vi "DMM Configuration - Update DMM Controls Items.vi"(6 "Measurement In":T2 caption="Function", 7 "Resolution in Digits Saved Value":dbl, 8 "error in (no error)":errorcluster, 11 "Measurement Controls Refs":T1) -> (0 "error out":errorcluster, 1 "Resolution in Digits Array Out":dbl[](array[numeric]), 2 "Resolution in Digits Index":i32)   [LabVIEW 2016, in "DMM-SWITCH-ScanList System Explorer.lvlib"]
doc: "Measurements, Range and Resolution in Digits original type definitions from the DMM driver were very old controls. In order to use System Controls to match our Custom Device guidelines this VI was necessary to populate the new System Controls with the data from the original Type Definitions."
uses:
  DMM-SWITCH-ScanList System Explorer.lvlib
  <instrlib>/niDMM/nidmm.llb/niDMM Resolution in Digits.ctl
  <instrlib>/niDMM/nidmm.llb/niDMM Function.ctl
panel:
  in  "Measurement Type Def":T2 caption="Function"
  in  "Resolution in Digits Type Def":T3=6.5 caption="Resolution In Digits Type Def" items=["3 1/2"=3.5, "4 1/2"=4.5, "5 1/2"=5.5, "6 1/2"=6.5, "7 1/2"=7.5]
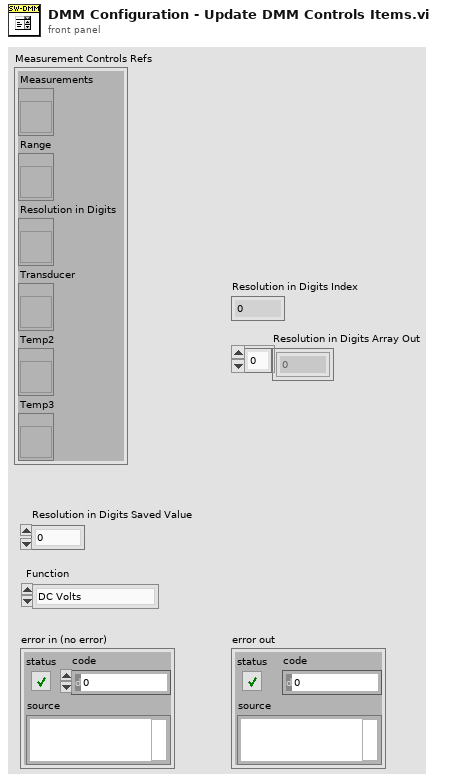
[diagram p1: front panel]
types:
  T1 = cluster{"Measurements":refnum<vi>, "Range":refnum<vi>, "Resolution in Digits":refnum<vi>, "Transducer":refnum<vi>, "Temp2":refnum<vi>, "Temp3":refnum<vi>}
  T2 = typedef "niDMM Function.ctl" = enum16{"DC Volts", "AC Volts", "DC Current", "AC Current", "2-wire Resistance", "4-wire Resistance", "Diode", "Frequency", "Period", "AC Volts DC Coupled", "Capacitance", "Inductance", "Temperature"}
  T3 = typedef "niDMM Resolution in Digits.ctl" = dbl
  T4 = typedef "LVStringsAndValuesArrayTypeDef_DBL.ctl" = cluster{"String":string, "Value":dbl}[]
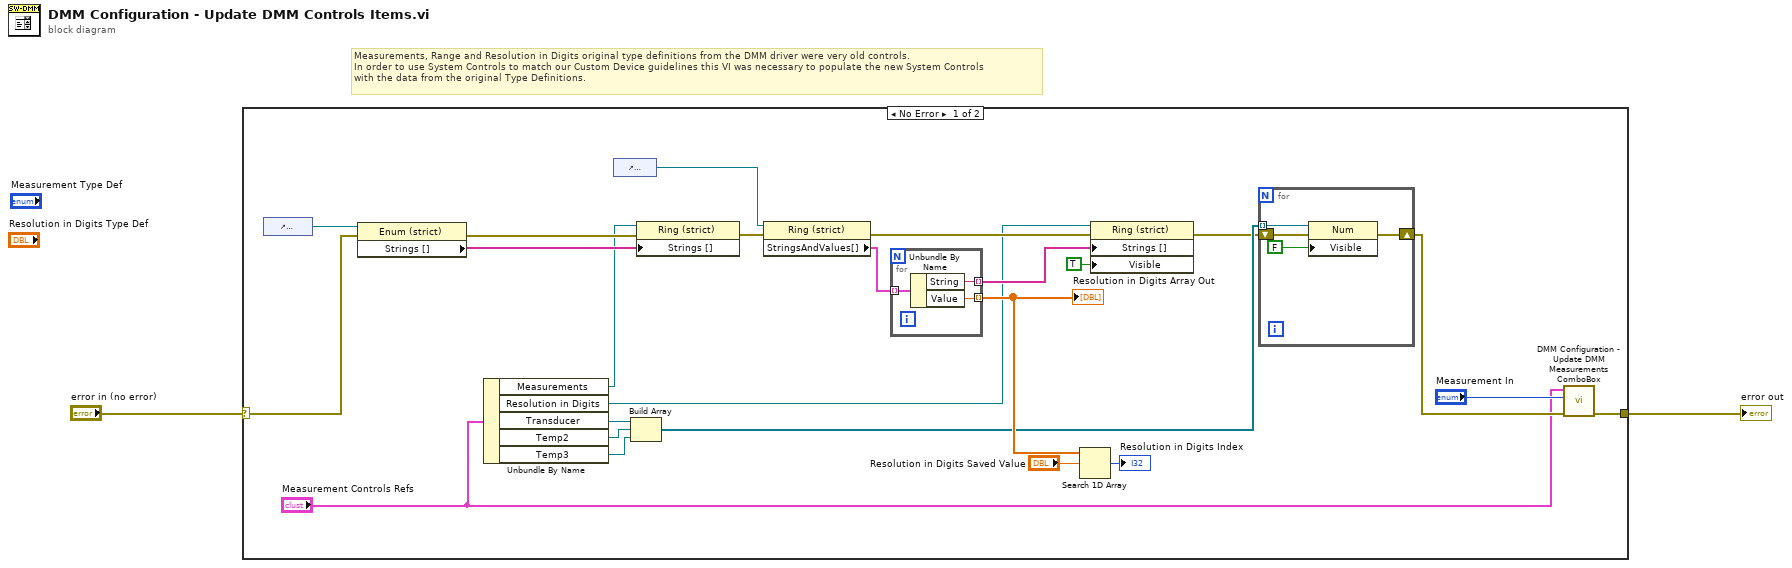
[diagram p0: block diagram]
diagram:
  # "Measurements, Range and Resolution in Digits original type definitions from the DMM driver were very old controls.\nIn order to use System Controls to match our Custom Device guidelines this VI was necessary to populate the new System Controls\nwith the data from the original Type Definitions."
  n1 = case shown="No Error" "error in (no error)" {
    selector: "error in (no error)" -> [w16 w34]
    tunnel: [w15 w34] -> w2
    frame No Error {
      n2 = control-ref of="Measurement Type Def"() -> (w4:refnum<vi>)
      n3 = property on="Property Node" class="Enum (strict)"(reference=w4, error in=w16) -> (error out=w25:errorcluster, "Strings []"=w26:string[])  [unwired: 1 out]
      n4 = Unbundle By Name("Measurement Controls Refs") -> ("Measurements"=w13:refnum<vi>, "Resolution in Digits"=w12:refnum<vi>, "Transducer"=w10:refnum<vi>, "Temp2"=w9:refnum<vi>, "Temp3"=w8:refnum<vi>)
      n5 = control-ref of="Resolution in Digits Type Def"() -> (w17:refnum<vi>)
      n6 = Build Array(w10, w9, w8) -> (w7:refnum<vi>[])
      n7 = property on="Property Node" class="Ring (strict)"(reference=w13, error in=w25, "Strings []"=w26) -> (error out=w22:errorcluster)  [unwired: 1 out]
      n8 = property on="Property Node" class="Ring (strict)"(reference=w17, error in=w22) -> (error out=w24:errorcluster, "StringsAndValues[]"=w23:T4)  [unwired: 1 out]
      n9 = for {
        tunnel: w23 -> [w33] mode=indexing
        tunnel: [w32] -> w21 mode=indexing
        tunnel: [w31] -> w19 mode=indexing
        n10 = Unbundle By Name(w33) -> ("String"=w32:string, "Value"=w31:dbl)
      }
      "Resolution in Digits Array Out" <- w19
      n11 = Search 1D Array(1D array=w19, element="Resolution in Digits Saved Value") -> (index of element=→"Resolution in Digits Index":i32)  [unwired: 1 in]
      n12 = property on="Property Node" class="Ring (strict)"(reference=w12, error in=w24, "Strings []"=w21, "Visible"=TRUE) -> (error out=w6:errorcluster)  [unwired: 1 out]
      n13 = for {
        tunnel: w7 -> [w29] mode=indexing
        shift-right: [w27] -> w5
        shift-left: w6 -> [w28]
        n14 = property on="Property Node" class="Num"(reference=w29, error in=w28, "Visible"=FALSE) -> (error out=w27:errorcluster)  [unwired: 1 out]
      }
      n15 = call "DMM Configuration - Update DMM Measurements ComboBox.vi"("error in (no error)"=w5, "Measurement In"="Measurement In", "Measurement Controls Refs In"="Measurement Controls Refs") -> ("error out"=w15:errorcluster)  [unwired: 5 in, 3 out]
    }
    frame Error {
    }
  }
  "error out" <- w2
